vi "close.vi"(8 "error in":errorcluster, 11 "Modbus Slave runtime in":refnum<class "Modbus Module runtime.lvclass">) -> (0 "error out":errorcluster)   [LabVIEW 2015, in "Modbus Module runtime.lvclass"]
doc: "Provides an interface for terminating a module instance. While this interface performs no operations, a child should close and deallocate any open references or memory.Platypus Framework 1.0.1.65\nNI Systems Engineering - National Instruments"
uses:
  <vilib>/NI/DCAF/Modules/modbus/module/execution/Modbus Module runtime.lvclass
  <vilib>/NI/DCAF/Modules/modbus/module/execution/Modbus Module runtime.lvclass/Modbus Module runtime.ctl
  <vilib>/NI/DCAF/Modules/modbus/module/execution/message to background process.ctl
  <vilib>/NI/DCAF/Modules/modbus/module/execution/command enum.ctl
  <vilib>/NI/Tag Bus/table/data table.ctl
  <vilib>/NI/DCAF/Modules/modbus/module/execution/modbus asynch.vi
  <vilib>/NI/Modbus Library/API/Modbus API.lvclass
  <vilib>/NI/Tag Bus/table/data table.lvlib
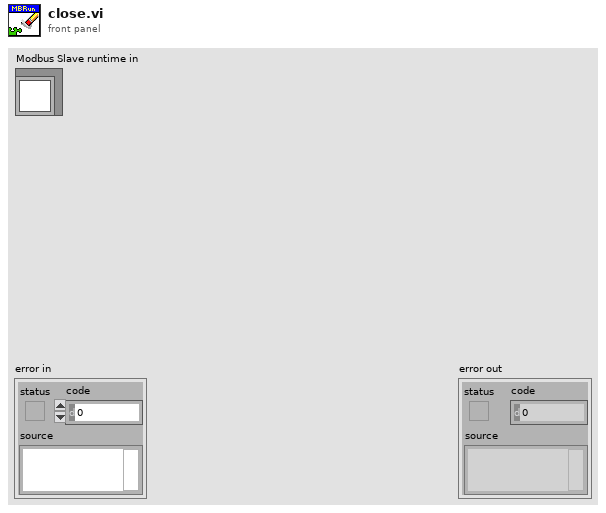
[diagram p1: front panel]
types:
  T1 = typedef "Modbus Module runtime.lvclass/asynch process references.ctl" = cluster{"commands":refnum<k33>, "input buffer":refnum<k33>, "output buffer":refnum<k33>, "asynch VI ref":variant, "original DVRs":refnum<data-value>[]}
  T2 = typedef "Modbus Module runtime.lvclass/message to background process.ctl" = cluster{"command enum":T3, "datapack":refnum<data-value>}
  T3 = typedef "Modbus Module runtime.lvclass/command enum.ctl" = enum16{"stop", "input", "output"}
  T4 = typedef "Modbus Module runtime.lvclass/response from background process.ctl" = cluster{"response enum":T5, "datapack":refnum<data-value>, "error code":i32}
  T5 = typedef "Modbus Module runtime.lvclass/response enum.ctl" = enum16{"exit", "return buffer", "error"}
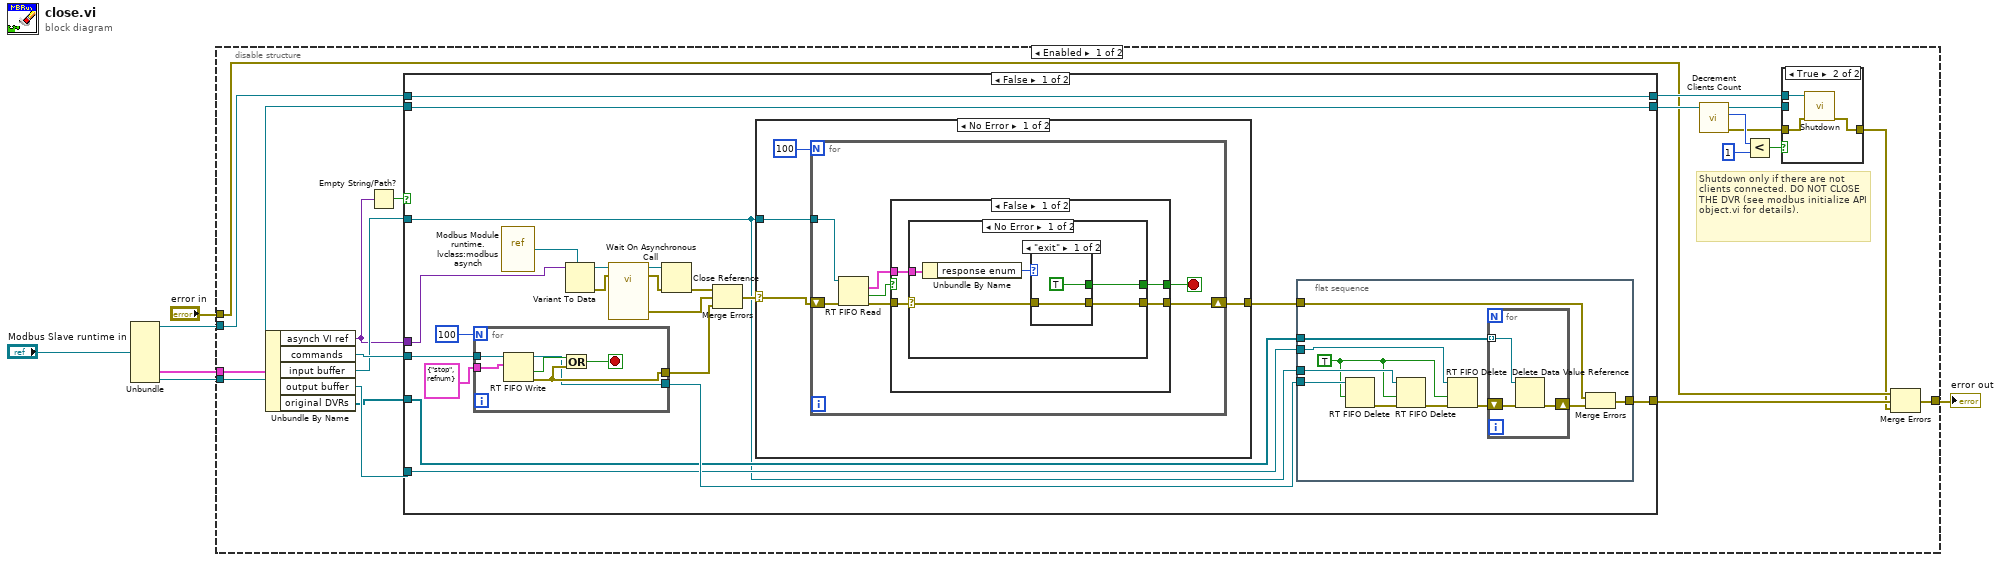
[diagram p0: block diagram]
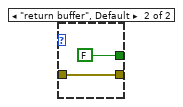
[diagram p3: hidden frame]
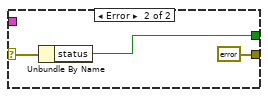
[diagram p4: hidden frame]
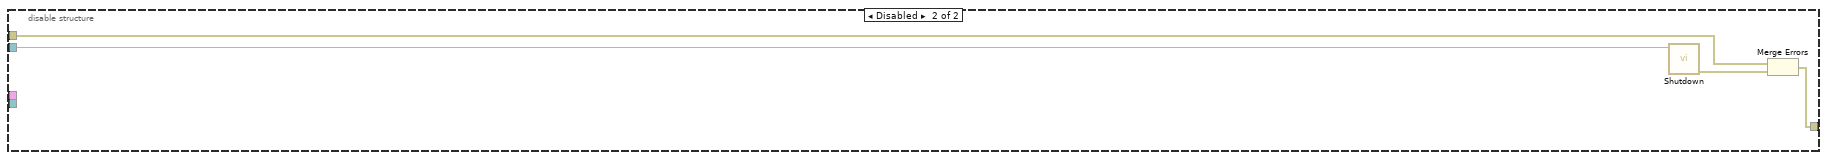
[diagram p8: hidden frame]
diagram:
  n1 = Unbundle("Modbus Slave runtime in") -> (w5:refnum<class "Modbus API.lvclass">, w4:T1, w1:refnum<data-value>)  [unwired: 5 out]
  n2 = disable-structure shown="Enabled" {
    disable-tunnel: w5 -> [w19 w105]
    disable-tunnel: w4 -> [w26 _]
    disable-tunnel: [w17 w107] -> w3
    disable-tunnel: "error in" -> [w9 w106]
    disable-tunnel: w1 -> [w16 _]
    frame Enabled {
      # "Shutdown only if there are not clients connected. DO NOT CLOSE THE DVR (see modbus initialize API object.vi for details)."
      n3 = Unbundle By Name(w26) -> ("asynch VI ref"=w21:variant, "commands"=w25:refnum<k33>, "input buffer"=w22:refnum<k33>, "output buffer"=w24:refnum<k33>, "original DVRs"=w23:refnum<data-value>[])
      n4 = Empty String/Path?(string/path=w21) -> (empty?=w20:bool)
      n5 = case shown="False" w20 {
        tunnel: w25 -> [w51 _]
        tunnel: w24 -> [w39 _]
        tunnel: w23 -> [w38 _]
        tunnel: w22 -> [w35 _]
        tunnel: [w34 _] -> w8
        tunnel: w21 -> [w33 _]
        tunnel: w19 -> [w32 w103]
        tunnel: [w32 w103] -> w18
        tunnel: w16 -> [w31 w102]
        tunnel: [w31 w102] -> w15
        frame False {
          n6 = for {
            N: 100 -> [_]
            tunnel: w51 -> [w101]
            tunnel: T2 {"command enum"=enum."stop", "datapack"=refnum} ("element") -> [w100]
            tunnel: [w97] -> w41
            tunnel: [w96] -> w40
            stop <- w98 stop-if-true
            n7 = RT FIFO Write(0:w101, 1:w100) -> (8:w96:refnum<k33>, 10:w99:bool, 11:w97:errorcluster)  [unwired: 3 in, 1 out]
            n8 = Or(x=w99, y=w97) -> (x .or. y?=w98:bool)
          }
          n9 = vi-ref "Modbus Module runtime.lvclass:modbus asynch.vi"() -> (w48:refnum<vi>)
          n10 = Variant To Data(type=w48, Variant=w33) -> (data=w47:refnum<vi>, error out=w46:errorcluster)  [unwired: 1 in]
          n11 = call-by-ref "Wait On Asynchronous Call"(reference=w47, error in=w46) -> (reference out=w44:refnum<vi>, error out=w45:errorcluster, 0:"error out"=w42:errorcluster)  [unwired: 11 in]
          n12 = Close Reference(reference=w44, error in (no error)=w45) -> (error out=w43:errorcluster)
          n13 = Merge Errors(w43, w42, w41) -> (w37:errorcluster)
          n14 = case shown="No Error" w37 {
            selector: w37 -> [w68 w95]
            tunnel: [w66 w95] -> w36
            tunnel: w35 -> [w67 _]
            frame No Error {
              n15 = for {
                N: 100 -> [_]
                shift-right: [w70] -> w66
                shift-left: w68 -> [w76]
                tunnel: w67 -> [w75]
                stop <- w72 stop-if-true
                n16 = RT FIFO Read(0:w75, 3:w76) -> (9:w74:T4, 10:w73:bool, 11:w71:errorcluster)  [unwired: 2 in, 2 out]
                n17 = case shown="False" w73 {
                  selector: w73 -> [_ w94]
                  tunnel: w74 -> [w80 _]
                  tunnel: [w77 w94] -> w72
                  tunnel: w71 -> [w79 w93]
                  tunnel: [w78 w93] -> w70
                  frame False {
                    n18 = case shown="No Error" w79 {
                      selector: w79 -> [w83 w92]
                      tunnel: w80 -> [w85 _]
                      tunnel: [w82 errorcluster {"status"=FALSE, "code"=0, "source"=""} ("error IO")] -> w78
                      tunnel: [w81 w91] -> w77
                      frame No Error {
                        n19 = Unbundle By Name(w85) -> ("response enum"=w84:T5)
                        n20 = case shown="\"exit\"" w84 {
                          tunnel: w83 -> [w86 w89]
                          tunnel: [w86 w89] -> w82
                          tunnel: [TRUE FALSE] -> w81
                          frame "exit" {
                          }
                          frame "return buffer", Default {
                          }
                        }
                      }
                      frame Error {
                        n21 = Unbundle By Name(w92) -> ("status"=w91:bool)
                      }
                    }
                  }
                  frame True {
                  }
                }
              }
            }
            frame Error {
            }
          }
          n22 = flat-sequence {
            tunnel: w40 -> [w62]
            tunnel: w39 -> [w61]
            tunnel: w38 -> [w60]
            tunnel: w36 -> [w59]
            tunnel: w35 -> [w58]
            tunnel: [w57] -> w34
            frame #0 {
              w53 = TRUE ("force destroy? (F)")
              n23 = RT FIFO Delete(0:w62, 2:w53) -> (11:w56:errorcluster)  [unwired: 1 in]
              n24 = RT FIFO Delete(0:w58, 2:w53, 3:w56) -> (11:w55:errorcluster)
              n25 = RT FIFO Delete(0:w61, 2:w53, 3:w55) -> (11:w52:errorcluster)
              n26 = for {
                tunnel: w60 -> [w65] mode=indexing
                shift-right: [w64] -> w54
                shift-left: w52 -> [w63]
                n27 = Delete Data Value Reference(data value reference=w65, error in=w63) -> (error out=w64:errorcluster)  [unwired: 1 out]
              }
              n28 = Merge Errors(w59, w54) -> (w57:errorcluster)
            }
          }
        }
        frame True {
        }
      }
      n29 = call <vilib>:"Decrement Clients Count.vi"("Data Value Reference in"=w15) -> ("error out"=w10:errorcluster, "Clients count"=w14:i32, "Data Value Reference out"=w11:refnum<data-value>)  [unwired: 8 in]
      n30 = Less?(x=w14, y=1) -> (x < y?=w12:bool)
      n31 = case shown="True" w12 {
        tunnel: w18 -> [_ w30]
        tunnel: w11 -> [_ _]
        tunnel: w10 -> [w27 w28]
        tunnel: [w27 w29] -> w7
        frame False {
        }
        frame True {
          n32 = call-dynamic "Shutdown.vi"("error in"=w28, "Modbus instance in"=w30) -> ("error out"=w29:errorcluster)  [unwired: 9 in]
        }
      }
      n33 = Merge Errors(w9, w8, w7) -> (w17:errorcluster)
    }
    frame Disabled {
      n34 = call-dynamic "Shutdown.vi"("Modbus instance in"=w105) -> ("error out"=w104:errorcluster)  [unwired: 10 in]
      n35 = Merge Errors(w106, w104) -> (w107:errorcluster)
    }
  }
  "error out" <- w3
